vi "Get Personality from SN.vi"(8 "error in (no error)":errorcluster, 11 "SN":string) -> (0 "error out":errorcluster, 3 "DB personality":T1)   [LabVIEW 2018, in "Personalities Tool.lvlib"]
doc: "This VI fetches the RIO personality from the Serianl Number."
uses:
  Personalities Tool.lvlib
  Controls/Personality Type.ctl
  <vilib>/Utility/config.llb/Read Key (String).vi
  <vilib>/Utility/config.llb/NI_LVConfig.lvlib
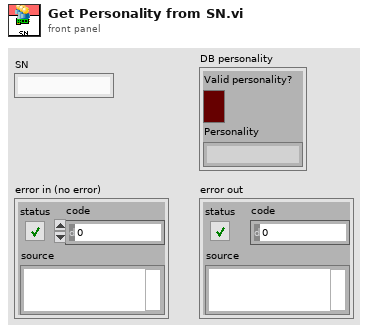
[diagram p1: front panel]
types:
  T1 = typedef "Personalities Tool.lvlib/Personality Type.ctl" = cluster{"Valid personality?":bool, "Personality":string}
  T2 = typedef "NI_LVConfig.lvlib/Config Data RefNum.ctl" = refnum<k1>
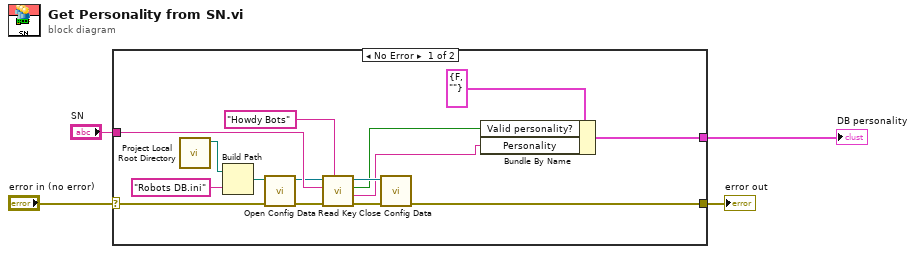
[diagram p0: block diagram]
diagram:
  n1 = case shown="No Error" "error in (no error)" {
    selector: "error in (no error)" -> [w17 w20]
    tunnel: [w19 _] -> w4
    tunnel: [w5 w20] -> w3
    tunnel: "SN" -> [w16 _]
    frame No Error {
      n2 = call "Project Local Root Directory.vi"() -> ("Code root's folder"=w12:path)  [unwired: 11 in]
      n3 = Build Path(base path=w12, name or relative path="Robots DB.ini") -> (appended path=w13:path)
      n4 = call <vilib>:"Open Config Data.vi"("error in (no error)"=w17, "configuration file path"=w13) -> ("error out"=w9:errorcluster, "refnum"=w8:T2)  [unwired: 7 in, 1 out]
      n5 = call-poly <vilib>:"Read Key.vi"("section"="Howdy Bots", "error in (no error)"=w9, "key"=w16, "refnum"=w8) -> ("error out"=w11:errorcluster, "value"=w6:string, "found?"=w7:bool, "refnum out"=w10:T2)  [unwired: 4 in]
      n6 = call <vilib>:"Close Config Data.vi"("error in (no error)"=w11, "refnum"=w10) -> ("error out"=w5:errorcluster)  [unwired: 8 in, 1 out]
      n7 = Bundle By Name(cluster=T1 {"Valid personality?"=FALSE, "Personality"=""} ("Cluster"), "Valid personality?"=w7, "Personality"=w6) -> (w19:T1)
    }
    frame Error {
    }
  }
  "DB personality" <- w4
  "error out" <- w3
